vi "Write Sorting Column.vi"(8 "nn (no error)":errorcluster, 10 "Sorting Column":i32, 11 "EngineTags in":refnum<class "Engine Mappings.lvclass">) -> (0 "error out":errorcluster, 3 "EngineTags out":refnum<class "Engine Mappings.lvclass">)   [LabVIEW 2013, in "PL Framework Configuration Tool.lvlib" / "Engine Mappings.lvclass"]
uses:
  Engine Mappings.lvclass
  Engine Mappings.lvclass/Engine Mappings.ctl
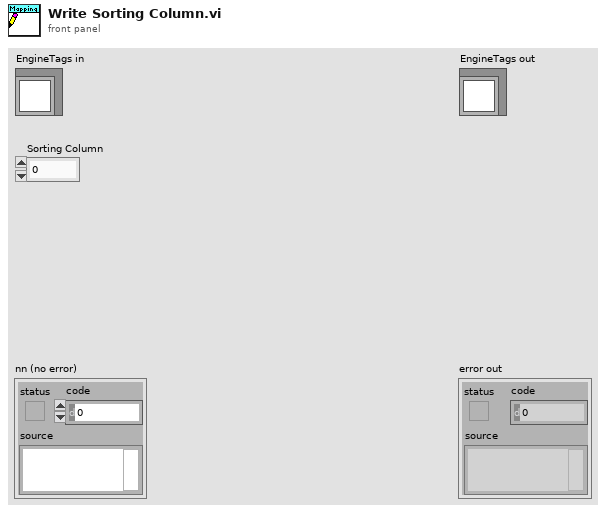
[diagram p1: front panel]
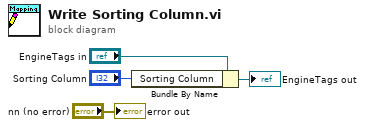
[diagram p0: block diagram]
diagram:
  n1 = Bundle By Name(cluster="EngineTags in", "Sorting Column"="Sorting Column") -> (→"EngineTags out":refnum<class "Engine Mappings.lvclass">)
  "error out" <- "nn (no error)"
